vi "VCL.vi"(8 "Stopp":bool, 10 "SLOT":i32=100 min=0 max=999 step=100 format="%03d", 11 "USB":i32) -> ()   [LabVIEW 2020]
doc: "This VI provides a GUI for VCL modules. It implements an abstract module interface, where callers provide the only necessary and sufficient information for callee modules via the datafields USB, SLOT and Stopp. All module intern information are handled hidden by the module. Thereby, a caller must not \"know\" about such internals."
panel:
  in  "Temperature":sgl caption="Temperature / °C" min=15 max=55 step=0.1 format="%.1g"
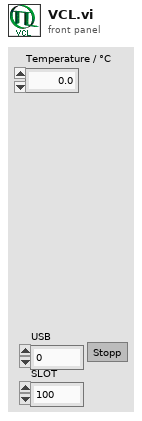
[diagram p1: front panel]
types:
  T1 = cluster{"MinTemperature":i32, "MaxTemperature":i32, "UserResolution":i32}
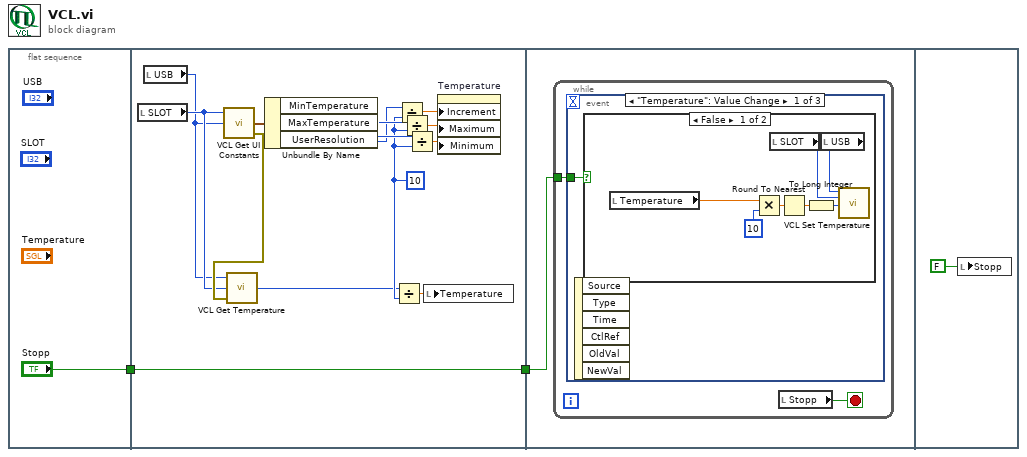
[diagram p0: block diagram]
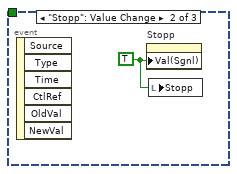
[diagram p3: hidden frame]
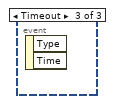
[diagram p4: hidden frame]
diagram:
  n1 = flat-sequence {
    tunnel: ["Stopp"] -> w1
    tunnel: [w13] -> w2
    tunnel: w1 -> [w13]
    tunnel: w2 -> [w18]
    frame #0 {
    }
    frame #1 {
      w5 = 10
      n2 = local read "SLOT"() -> (w15:i32)
      n3 = local read "USB"() -> (w14:i32)
      n4 = call "VCL Get UI Constants.vi"("DevIdx"=w14, "SlotId"=w15) -> ("error out"=w17:errorcluster, "VCL UI Constants"=w16:T1)  [unwired: 1 in, 1 out]
      n5 = call "VCL Get Temperature.vi"("error in (no error)"=w17, "SlotId"=w15, "DevIdx"=w14) -> ("Temperature / 0.1 °C"=w4:i32)  [unwired: 2 out]
      n6 = Unbundle By Name(w16) -> ("MinTemperature"=w9:i32, "MaxTemperature"=w8:i32, "UserResolution"=w7:i32)
      n7 = Divide(x=w4, y=w5) -> (x/y=w6:dbl)
      n8 = Divide(x=w7, y=w5) -> (x/y=w10:dbl)
      n9 = Divide(x=w8, y=w5) -> (x/y=w11:dbl)
      n10 = Divide(x=w9, y=w5) -> (x/y=w12:dbl)
      n11 = local write "Temperature"(w6) -> ()
      n12 = property on="Temperature" class="DigNum (strict)"("Increment"=w10, "Maximum"=w11, "Minimum"=w12) -> ()  [unwired: 2 in, 2 out]
    }
    frame #2 {
      n13 = while {
        tunnel: w18 -> [w19]
        stop <- w20 stop-if-true
        n14 = event shown="[0] \"Temperature\": Value Change" {
          selector: _ -> [_ _ _]
          dyn-events: _ -> [_ _ _]
          timeout: _ -> [_ _ _]
          tunnel: w19 -> [w21 _ _]
          event "Temperature": Value Change {
            n15 = event-data() -> ()  [unwired: 1 in, 6 out]
            n16 = case shown="False" w21 {
              frame False {
                n17 = local read "Temperature"() -> (w22:sgl)
                n18 = Multiply(x=w22, y=10) -> (x*y=w23:sgl)
                n19 = local read "SLOT"() -> (w27:i32)
                n20 = Round To Nearest(number=w23) -> (nearest integer value=w25:sgl)
                n21 = To Long Integer(number=w25) -> (32bit integer=w26:i32)
                n22 = local read "USB"() -> (w28:i32)
                n23 = call "VCL Set Temperature.vi"("Temperature"=w26, "SlotId"=w27, "DevIdx"=w28) -> ()  [unwired: 1 in, 2 out]
              }
              frame True {
              }
            }
          }
          event "Stopp": Value Change {
            w29 = TRUE ("Value (Signaling)")
            n24 = event-data() -> ()  [unwired: 1 in, 6 out]
            n25 = property on="Stopp" class="Bool (strict)"("Val(Sgnl)"=w29) -> ()  [unwired: 2 in, 2 out]
            n26 = local write "Stopp"(w29) -> ()
          }
          event Timeout {
            n27 = event-data() -> ()  [unwired: 1 in, 2 out]
          }
        }
        n28 = local read "Stopp"() -> (w20:bool)
      }
    }
    frame #3 {
      n29 = local write "Stopp"(FALSE ("Stopp")) -> ()
    }
  }
